vi "load_ent_log.vi"   [LabVIEW 2012]
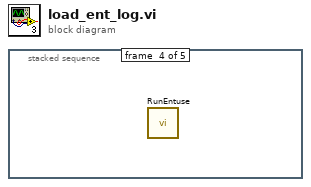
[diagram p0: block diagram]
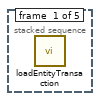
[diagram p2: hidden frame]
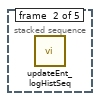
[diagram p3: hidden frame]
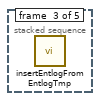
[diagram p4: hidden frame]
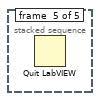
[diagram p5: hidden frame]
diagram:
  n1 = stacked-sequence {
    frame #0 {
      n2 = call "loadEntityTransaction.vi"() -> ()  [unwired: 12 in]
    }
    frame #1 {
      n3 = call "updateEnt_logHistSeq.vi"() -> ()  [unwired: 12 in]
    }
    frame #2 {
      n4 = call "insertEntlogFromEntlogTmp.vi"() -> ()  [unwired: 12 in]
    }
    frame #3 {
      n5 = call "RunEntuse.vi"() -> ()  [unwired: 12 in]
    }
    frame #4 {
      n6 = Quit LabVIEW() -> ()  [unwired: 1 in]
    }
  }
